vi "CRYDataView Add Graph VI.vi"(4 "DataView Idx":i32, 6 "Graph Main VIRef In":refnum<vi>, 7 "isFirstPanel":bool, 8 "Queue Name":string, 9 "GraphType":string="XY", 10 "panel_index":i32, 11 "Panel Ref In":refnum<vi>) -> (3 "bResult":bool)   [LabVIEW 2013]
uses:
  CRYNew View Global.vi
  SubVI/CRYData View Global.vi
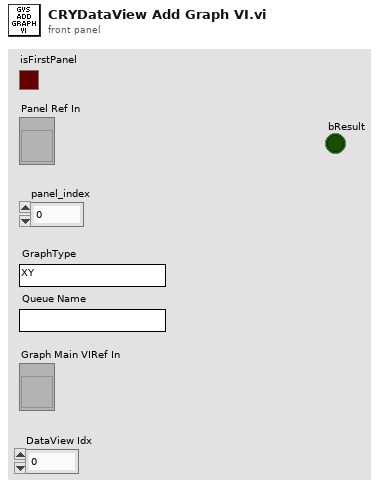
[diagram p1: front panel]
types:
  T1 = typedef "Graph Main Info Cluster.ctl" = cluster{"Selected_BarIdx":i32, "Selected_PanelIdx":i32, "Graph Main VIRef":refnum<vi>, "ToolBarClick":bool, "Spliter Ref Array":refnum<vi>[], "Panel Ref Array":refnum<vi>[], "Spliter_matrix":i32[][], "Panel_matrix":i32[][], "child_spliterIdx_matrix":i32[][], "split_pos_matrix":i32[][], "Title State":bool, "sQueueName":string, "Frame nID":i32, "Graph VIRef Array":cluster{"Graph VIRef":refnum<vi>, "Panel Idx":i32, "Frame VIRef":refnum<vi>, "Icon Ring":i32, "Graph Type":string}[], "View Type":string}
  T2 = cluster{"Graph VIRef":refnum<vi>, "Panel Idx":i32, "Frame VIRef":refnum<vi>, "Icon Ring":i32, "Graph Type":string}
  T3 = typedef "LVRectTypeDef.ctl" = cluster{"Left":i16, "Top":i16, "Right":i16, "Bottom":i16}
  T4 = typedef "CRYGraph Event.ctl" = cluster{"EvenName":string, "TitleName":string, "GraphName":string, "GraphType":string, "Data":variant, "Queue Name":string, "DataView Number":i32}
  T5 = cluster{"Graph VIRef":refnum<vi>, "Panel Idx":i32, "Frame VIRef":refnum<vi>, "Icon Ring":i32, "Graph Type":string}[]
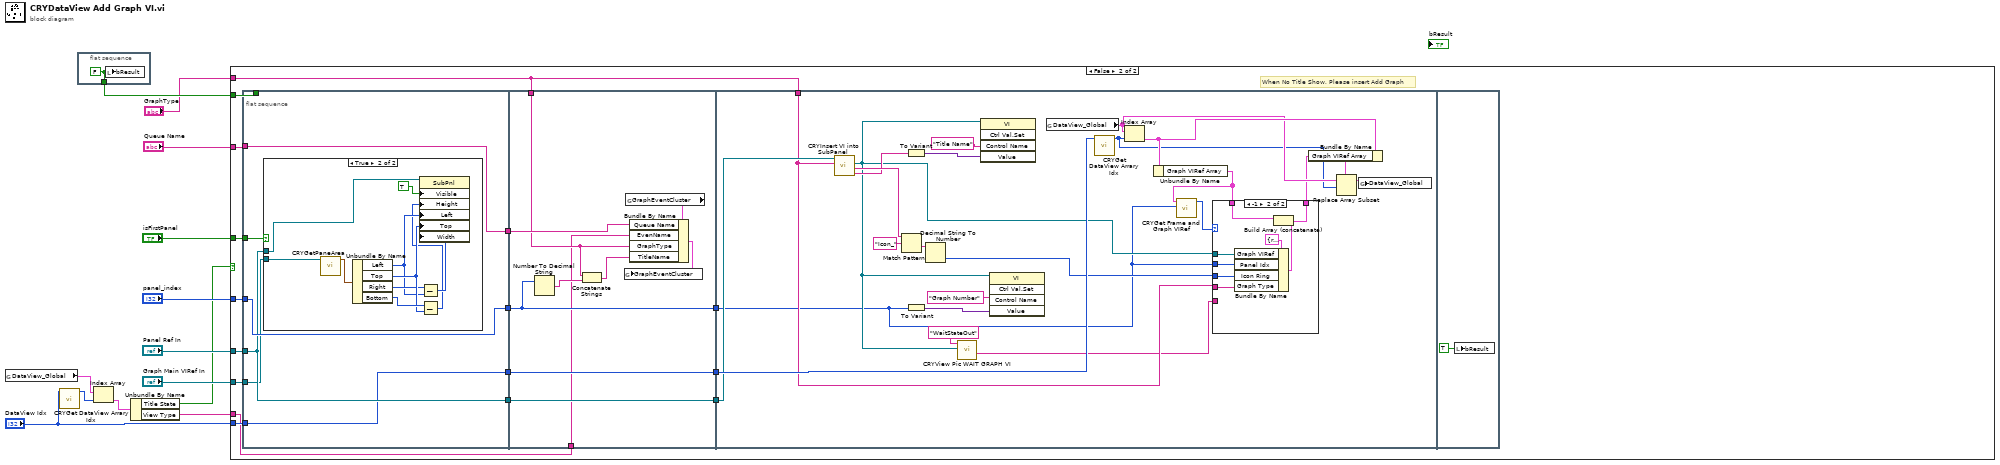
[diagram p0: block diagram]
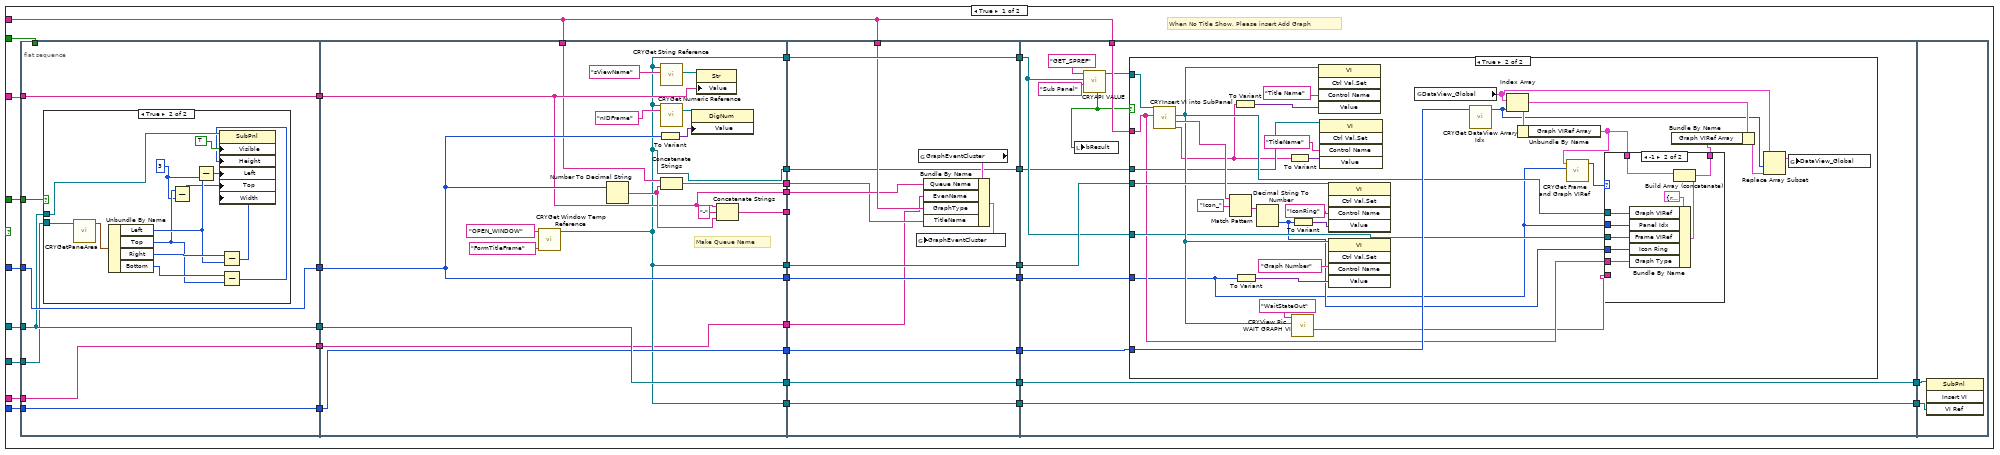
[diagram p2: hidden frame]
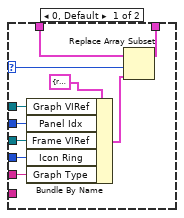
[diagram p5: hidden frame]
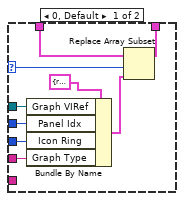
[diagram p7: hidden frame]
diagram:
  n1 = global read "CRYNew View Global.vi" "DataView_Global"() -> (w5:T1[])
  n2 = call "CRYGet DataView Arrary Idx.vi"("DataView Idx In"="DataView Idx") -> ("DataView Arrary Idx out"=w4:i32)  [unwired: 10 in]
  n3 = flat-sequence {
    tunnel: [w14] -> w8
    frame #0 {
      w14 = FALSE ("bResult")
      n4 = local write "bResult"(w14) -> ()
    }
  }
  n5 = Index Array(array=w5, index=w4) -> (element=w3:T1)
  n6 = Unbundle By Name(w3) -> ("Title State"=w2:bool, "View Type"=w1:string)
  n7 = case shown="False" w2 {
    tunnel: "panel_index" -> [w25 w176]
    tunnel: "Panel Ref In" -> [w24 w175]
    tunnel: "Queue Name" -> [w23 w174]
    tunnel: "Graph Main VIRef In" -> [w22 w173]
    tunnel: "isFirstPanel" -> [w21 w172]
    tunnel: w8 -> [w20 w171]
    tunnel: "DataView Idx" -> [w19 w170]
    tunnel: "GraphType" -> [w18 w169]
    tunnel: w1 -> [w16 w164]
    frame True {
      # "When No Title Show, Please insert Add Graph"
      n8 = flat-sequence {
        tunnel: w24 -> [w52]
        tunnel: w23 -> [w54]
        tunnel: w25 -> [w55]
        tunnel: [w55] -> w48
        tunnel: [w54] -> w47
        tunnel: [w52] -> w46
        tunnel: w22 -> [w51]
        tunnel: w21 -> [w53]
        tunnel: w20 -> [_]
        tunnel: [w50] -> w45
        tunnel: w19 -> [w50]
        tunnel: [w49] -> w17
        tunnel: w16 -> [w49]
        tunnel: [w70] -> w44
        tunnel: w48 -> [w75]
        tunnel: w47 -> [w73]
        tunnel: w46 -> [w74]
        tunnel: [w79] -> w43
        tunnel: [w76] -> w42
        tunnel: [w70] -> w41
        tunnel: [w75] -> w40
        tunnel: [w74] -> w39
        tunnel: [w70] -> w38
        tunnel: [w73] -> w37
        tunnel: w45 -> [w72]
        tunnel: [w72] -> w36
        tunnel: w18 -> [w71]
        tunnel: [w70] -> w35
        tunnel: w17 -> [w69]
        tunnel: [w69] -> w15
        tunnel: w44 -> [w99]
        tunnel: [w99] -> w34
        tunnel: w18 -> [w96]
        tunnel: w43 -> [w89]
        tunnel: w42 -> [_]
        tunnel: [w95] -> w33
        tunnel: w41 -> [w95]
        tunnel: [w94] -> w32
        tunnel: w40 -> [w94]
        tunnel: [w93] -> w31
        tunnel: w39 -> [w93]
        tunnel: w38 -> [w92]
        tunnel: [w92] -> w30
        tunnel: w37 -> [w91]
        tunnel: [w90] -> w29
        tunnel: w36 -> [w90]
        tunnel: [w88] -> w28
        tunnel: w35 -> [w88]
        tunnel: w15 -> [w87]
        tunnel: w34 -> [w101]
        tunnel: w18 -> [w111]
        tunnel: w33 -> [w106]
        tunnel: w32 -> [w105]
        tunnel: [w104] -> w27
        tunnel: w31 -> [w104]
        tunnel: w30 -> [w103]
        tunnel: [w103] -> w26
        tunnel: w29 -> [w102]
        tunnel: w28 -> [w100]
        tunnel: w27 -> [w163]
        tunnel: w26 -> [w162]
        frame #0 {
          n9 = case shown="True" w53 {
            tunnel: w52 -> [_ w62]
            tunnel: w51 -> [_ w61]
            frame False {
            }
            frame True {
              w56 = i16 3 ("y")
              n10 = call "CRYGetPaneArea.vi"("vi reference"=w61) -> ("Content Area Rect"=w67:T3)  [unwired: 10 in]
              n11 = Unbundle By Name(w67) -> ("Left"=w64:i16, "Top"=w57:i16, "Right"=w65:i16, "Bottom"=w66:i16)
              n12 = Subtract(x=w57, y=w56) -> (x-y=w58:i16)
              n13 = Subtract(x=w64, y=w56) -> (x-y=w60:i16)
              n14 = Subtract(x=w65, y=w64) -> (x-y=w63:i16)
              n15 = Subtract(x=w66, y=w57) -> (x-y=w59:i16)
              n16 = property class="SubPnl"(reference=w62, "Visible"=TRUE, "Height"=w59, "Left"=w60, "Top"=w58, "Width"=w63) -> ()  [unwired: 1 in, 2 out]
            }
          }
        }
        frame #1 {
          # "Make Queue Name"
          n17 = call "CRYGet Window Temp Reference.vi"("sWindowName"="FormTitleFrame", "sAction"="OPEN_WINDOW") -> ("pVIRef_Out"=w70:refnum<vi>)  [unwired: 5 in, 4 out]
          n18 = Number To Decimal String(number=w75) -> (decimal integer string=w77:string)  [unwired: 1 in]
          n19 = To Variant(anything=w75) -> (Variant=w83:variant)
          n20 = call "CRYGet String Reference.vi"("Label Name"="sViewName", "VI Refnum"=w70) -> ("String Ref Out"=w85:refnum<vi>)  [unwired: 7 in, 2 out]
          n21 = call "CRYGet Numeric Reference.vi"("Label Name"="nIDFrame", "VI Refnum"=w70) -> ("Numeric Ref Out"=w84:refnum<vi>)  [unwired: 7 in, 2 out]
          n22 = Concatenate Strings(w71, w77) -> (w79:string)
          n23 = property class="DigNum"(reference=w84, "Value"=w83) -> ()  [unwired: 1 in, 2 out]
          n24 = property class="Str"(reference=w85, "Value"=w73) -> ()  [unwired: 1 in, 2 out]
          n25 = Concatenate Strings(w73, "-" ("string"), w77) -> (w76:string)
        }
        frame #2 {
          n26 = global read "CRYData View Global.vi" "GraphEventCluster"() -> (w98:T4)
          n27 = Bundle By Name(cluster=w98, "Queue Name"=w91, "EvenName"=w87, "GraphType"=w96, "TitleName"=w89) -> (w97:T4)
          n28 = global write "CRYData View Global.vi" "GraphEventCluster"(w97) -> ()
        }
        frame #3 {
          n29 = call "CRYAPI VALUE.vi"("sControlName"="Sub Panel", "pVIRef"=w101, "sAction"="GET_SPREF") -> ("pSPRef"=w108:refnum<vi>, "bResult"=w107:bool)  [unwired: 2 in, 5 out]
          n30 = local write "bResult"(w107) -> ()
          n31 = case shown="True" w107 {
            tunnel: w111 -> [_ w116]
            tunnel: w108 -> [_ w142]
            tunnel: w106 -> [_ w136]
            tunnel: w105 -> [_ w114]
            tunnel: w102 -> [_ w132]
            tunnel: w101 -> [_ w124]
            tunnel: w100 -> [_ w121]
            frame False {
            }
            frame True {
              n32 = call "CRYInsert VI into SubPanel.vi"("WindowType"=w116, "SubPanel Ref"=w142) -> ("WindowName"=w118:string, "Icon Out"=w137:string, "VI Ref Out"=w125:refnum<vi>)  [unwired: 6 in, 1 out]
              n33 = Match Pattern(string=w137, regular expression="Icon_") -> (after substring=w141:string)  [unwired: 1 in, 3 out]
              n34 = To Variant(anything=w118) -> (Variant=w123:variant)
              n35 = To Variant(anything=w114) -> (Variant=w134:variant)
              n36 = Decimal String To Number(string=w141) -> (number=w117:i32)  [unwired: 2 in, 1 out]
              n37 = To Variant(anything=w118) -> (Variant=w120:variant)
              n38 = call "CRYView Pic WAIT GRAPH VI.vi"("vi reference"=w125, "sAction"="WaitStateOut") -> ("sData_Out"=w112:string)  [unwired: 9 in]
              n39 = To Variant(anything=w117) -> (Variant=w138:variant)
              n40 = invoke class="VI" method="Ctrl Val.Set"(reference=w125, "Control Name"="Title Name" ("Label Name"), "Value"=w123) -> ()  [unwired: 2 in, 5 out]
              n41 = invoke class="VI" method="Ctrl Val.Set"(reference=w121, "Control Name"="TitleName" ("Label Name"), "Value"=w120) -> ()  [unwired: 2 in, 5 out]
              n42 = invoke class="VI" method="Ctrl Val.Set"(reference=w136, "Control Name"="IconRing", "Value"=w138) -> ()  [unwired: 2 in, 5 out]
              n43 = invoke class="VI" method="Ctrl Val.Set"(reference=w125, "Control Name"="Graph Number", "Value"=w134) -> ()  [unwired: 2 in, 5 out]
              n44 = global read "CRYNew View Global.vi" "DataView_Global"() -> (w129:T1[])
              n45 = call "CRYGet DataView Arrary Idx.vi"("DataView Idx In"=w132) -> ("DataView Arrary Idx out"=w128:i32)  [unwired: 10 in]
              n46 = Index Array(array=w129, index=w128) -> (element=w131:T1)
              n47 = Unbundle By Name(w131) -> ("Graph VIRef Array"=w115:T5)
              n48 = call "CRYGet Frame and Graph VIRef.vi"("Panel Idx"=w114, "Graph VIRef Array"=w115) -> ("Graph VIRef Array Index"=w113:i32)  [unwired: 5 in, 4 out]
              n49 = case shown="-1" w113 {
                selector: w113 -> [w150 _]
                tunnel: w115 -> [w152 w161]
                tunnel: [w151 w159] -> w130
                tunnel: w125 -> [w149 w158]
                tunnel: w114 -> [w148 w157]
                tunnel: w124 -> [w147 w156]
                tunnel: w117 -> [w146 w155]
                tunnel: w116 -> [w145 w153]
                tunnel: w112 -> [_ _]
                frame 0, Default {
                  n50 = Bundle By Name(cluster=T2 {"Graph VIRef"=refnum, "Panel Idx"=0, "Frame VIRef"=refnum, "Icon Ring"=0, "Graph Type"=""} ("element"), "Graph VIRef"=w149, "Panel Idx"=w148, "Frame VIRef"=w147, "Icon Ring"=w146, "Graph Type"=w145) -> (w143:T2)
                  n51 = Replace Array Subset(array=w152, new element=w143, index=w150) -> (w151:T5)
                }
                frame -1 {
                  n52 = Bundle By Name(cluster=T2 {"Graph VIRef"=refnum, "Panel Idx"=0, "Frame VIRef"=refnum, "Icon Ring"=0, "Graph Type"=""} ("element"), "Graph VIRef"=w158, "Panel Idx"=w157, "Frame VIRef"=w156, "Icon Ring"=w155, "Graph Type"=w153) -> (w160:T2)
                  n53 = Build Array (concatenate)(w161, w160) -> (w159:T5)
                }
              }
              n54 = Bundle By Name(cluster=w131, "Graph VIRef Array"=w130) -> (w127:T1)
              n55 = Replace Array Subset(array=w129, new element=w127, index=w128) -> (w126:T1[])
              n56 = global write "CRYNew View Global.vi" "DataView_Global"(w126) -> ()
            }
          }
        }
        frame #4 {
          n57 = invoke class="SubPnl" method="Insert VI"(reference=w163, "VI Ref"=w162) -> ()  [unwired: 2 in, 4 out]
        }
      }
    }
    frame False {
      # "When No Title Show, Please insert Add Graph"
      n58 = flat-sequence {
        tunnel: w175 -> [w182]
        tunnel: w174 -> [w184]
        tunnel: w176 -> [w185]
        tunnel: [w185] -> w168
        tunnel: [w184] -> w167
        tunnel: [w182] -> w166
        tunnel: w173 -> [w181]
        tunnel: w172 -> [w183]
        tunnel: w171 -> [_]
        tunnel: [w180] -> w165
        tunnel: w170 -> [w180]
        tunnel: w169 -> [w199]
        tunnel: [w198] -> w179
        tunnel: w168 -> [w198]
        tunnel: [w203] -> w178
        tunnel: w166 -> [w203]
        tunnel: w167 -> [w202]
        tunnel: [w201] -> w177
        tunnel: w165 -> [w201]
        tunnel: w164 -> [w196]
        tunnel: w169 -> [w210]
        tunnel: w179 -> [w207]
        tunnel: w178 -> [w228]
        tunnel: w177 -> [w229]
        frame #0 {
          n59 = case shown="True" w183 {
            tunnel: w182 -> [_ w187]
            tunnel: w181 -> [_ w186]
            frame False {
            }
            frame True {
              n60 = call "CRYGetPaneArea.vi"("vi reference"=w186) -> ("Content Area Rect"=w194:T3)  [unwired: 10 in]
              n61 = Unbundle By Name(w194) -> ("Left"=w190:i16, "Top"=w192:i16, "Right"=w191:i16, "Bottom"=w193:i16)
              n62 = Subtract(x=w191, y=w190) -> (x-y=w189:i16)
              n63 = Subtract(x=w193, y=w192) -> (x-y=w188:i16)
              n64 = property class="SubPnl"(reference=w187, "Visible"=TRUE, "Height"=w188, "Left"=w190, "Top"=w192, "Width"=w189) -> ()  [unwired: 1 in, 2 out]
            }
          }
        }
        frame #1 {
          n65 = Number To Decimal String(number=w198) -> (decimal integer string=w200:string)  [unwired: 1 in]
          n66 = Concatenate Strings(w199, w200) -> (w197:string)
          n67 = global read "CRYData View Global.vi" "GraphEventCluster"() -> (w205:T4)
          n68 = Bundle By Name(cluster=w205, "Queue Name"=w202, "EvenName"=w196, "GraphType"=w199, "TitleName"=w197) -> (w204:T4)
          n69 = global write "CRYData View Global.vi" "GraphEventCluster"(w204) -> ()
        }
        frame #2 {
          n70 = call "CRYInsert VI into SubPanel.vi"("WindowType"=w210, "SubPanel Ref"=w228) -> ("WindowName"=w214:string, "Icon Out"=w225:string, "VI Ref Out"=w212:refnum<vi>)  [unwired: 6 in, 1 out]
          n71 = Match Pattern(string=w225, regular expression="Icon_") -> (after substring=w227:string)  [unwired: 1 in, 3 out]
          n72 = To Variant(anything=w214) -> (Variant=w216:variant)
          n73 = To Variant(anything=w207) -> (Variant=w223:variant)
          n74 = Decimal String To Number(string=w227) -> (number=w211:i32)  [unwired: 2 in, 1 out]
          n75 = call "CRYView Pic WAIT GRAPH VI.vi"("vi reference"=w212, "sAction"="WaitStateOut") -> ("sData_Out"=w206:string)  [unwired: 9 in]
          n76 = invoke class="VI" method="Ctrl Val.Set"(reference=w212, "Control Name"="Title Name" ("Label Name"), "Value"=w216) -> ()  [unwired: 2 in, 5 out]
          n77 = invoke class="VI" method="Ctrl Val.Set"(reference=w212, "Control Name"="Graph Number", "Value"=w223) -> ()  [unwired: 2 in, 5 out]
          n78 = global read "CRYNew View Global.vi" "DataView_Global"() -> (w220:T1[])
          n79 = call "CRYGet DataView Arrary Idx.vi"("DataView Idx In"=w229) -> ("DataView Arrary Idx out"=w219:i32)  [unwired: 10 in]
          n80 = Index Array(array=w220, index=w219) -> (element=w221:T1)
          n81 = Unbundle By Name(w221) -> ("Graph VIRef Array"=w208:T5)
          n82 = call "CRYGet Frame and Graph VIRef.vi"("Panel Idx"=w207, "Graph VIRef Array"=w208) -> ("Graph VIRef Array Index"=w213:i32)  [unwired: 5 in, 4 out]
          n83 = case shown="-1" w213 {
            selector: w213 -> [w236 _]
            tunnel: w208 -> [w238 w246]
            tunnel: [w237 w244] -> w209
            tunnel: w212 -> [w235 w243]
            tunnel: w207 -> [w234 w242]
            tunnel: w211 -> [w233 w239]
            tunnel: w210 -> [w232 w240]
            tunnel: w206 -> [_ _]
            frame 0, Default {
              n84 = Bundle By Name(cluster=T2 {"Graph VIRef"=refnum, "Panel Idx"=0, "Frame VIRef"=refnum, "Icon Ring"=0, "Graph Type"=""} ("element"), "Graph VIRef"=w235, "Panel Idx"=w234, "Icon Ring"=w233, "Graph Type"=w232) -> (w230:T2)
              n85 = Replace Array Subset(array=w238, new element=w230, index=w236) -> (w237:T5)
            }
            frame -1 {
              n86 = Bundle By Name(cluster=T2 {"Graph VIRef"=refnum, "Panel Idx"=0, "Frame VIRef"=refnum, "Icon Ring"=0, "Graph Type"=""} ("element"), "Graph VIRef"=w243, "Panel Idx"=w242, "Icon Ring"=w239, "Graph Type"=w240) -> (w245:T2)
              n87 = Build Array (concatenate)(w246, w245) -> (w244:T5)
            }
          }
          n88 = Bundle By Name(cluster=w221, "Graph VIRef Array"=w209) -> (w218:T1)
          n89 = Replace Array Subset(array=w220, new element=w218, index=w219) -> (w217:T1[])
          n90 = global write "CRYNew View Global.vi" "DataView_Global"(w217) -> ()
        }
        frame #3 {
          n91 = local write "bResult"(TRUE ("bResult")) -> ()
        }
      }
    }
  }
